vi "Path Testing.vi"() -> ()   [LabVIEW 2020]
panel:
  out "Shared Data Dir path":path
  out "Default volume path":path
  out "Default path":path
  out "Application volume path":path
  out "Application path":path
  out "Temp volume path":path
  out "Temp path":path
  out "VI Lib volume path":path
  out "VI LIb path":path
  out "VI path":path
  out "VI volume path":path
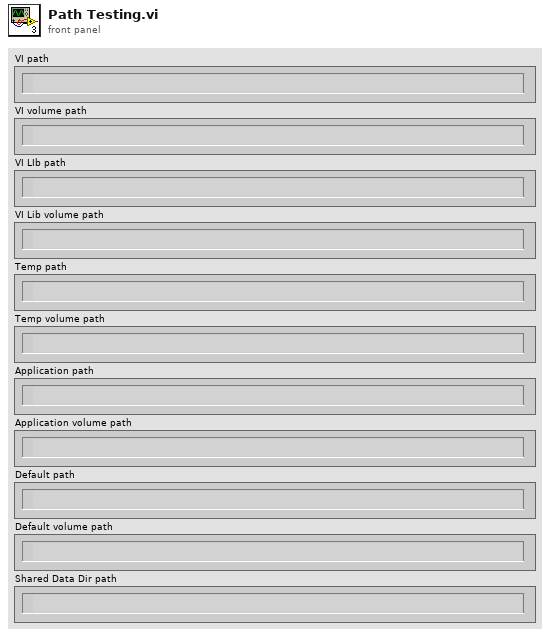
[diagram p1: front panel]
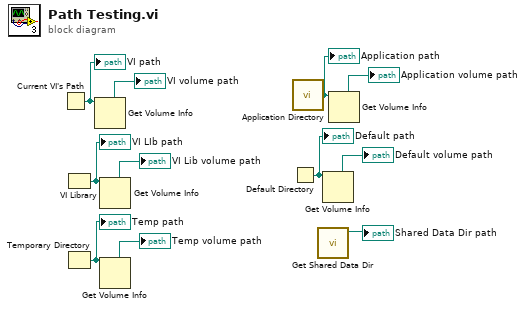
[diagram p0: block diagram]
diagram:
  n1 = Current VI's Path() -> (path=w11:path)
  "VI path" <- w11
  n2 = VI Library() -> (path=w2:path)
  "VI LIb path" <- w2
  n3 = Temporary Directory() -> (w3:path)
  "Temp path" <- w3
  n4 = Get Volume Info(11:w11) -> (5:→"VI volume path":path)  [unwired: 1 in, 5 out]
  n5 = Get Volume Info(11:w2) -> (5:→"VI Lib volume path":path)  [unwired: 1 in, 5 out]
  n6 = Get Volume Info(11:w3) -> (5:→"Temp volume path":path)  [unwired: 1 in, 5 out]
  n7 = Default Directory() -> (w5:path)
  "Default path" <- w5
  n8 = call <vilib>:"Application Directory.vi"() -> ("Application Directory"=w4:path)
  "Application path" <- w4
  n9 = call "Get Shared Data Dir.vi"() -> ("Data Directory Path"=→"Shared Data Dir path":path)  [unwired: 2 in, 1 out]
  n10 = Get Volume Info(11:w5) -> (5:→"Default volume path":path)  [unwired: 1 in, 5 out]
  n11 = Get Volume Info(11:w4) -> (5:→"Application volume path":path)  [unwired: 1 in, 5 out]
